vi "AssertFalse.vi"(7 "Message (\"\")":string, 8 "error in (no error)":errorcluster, 10 "Condition":bool) -> (0 "error out":errorcluster, 2 "Result":bool)   [LabVIEW 2019, in "Assertion.lvlib"]
doc: "Asserts that a condition is <B>false</B>. Does nothing if an error occurred before this node runs. Returns an error if the assertion failed. Optionally adds a message to the error message if the assertion failed."
uses:
  Assertion.lvlib
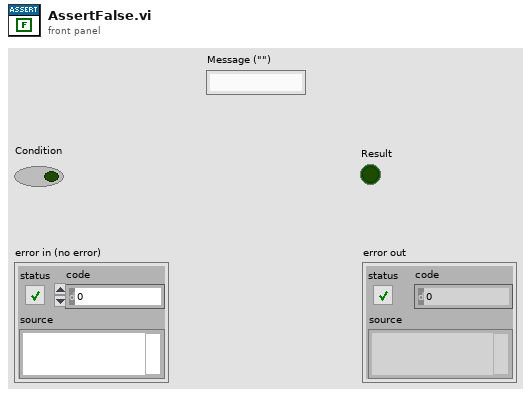
[diagram p1: front panel]
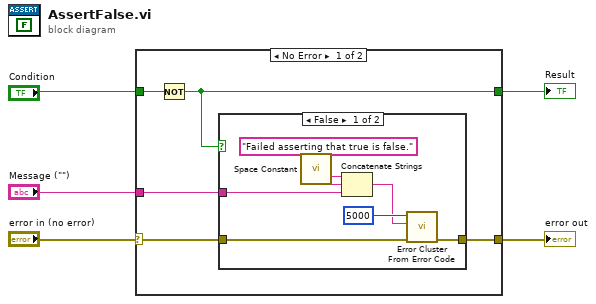
[diagram p0: block diagram]
diagram:
  n1 = case shown="No Error" "error in (no error)" {
    selector: "error in (no error)" -> [w9 w19]
    tunnel: "Condition" -> [w10 _]
    tunnel: [w7 _] -> w1
    tunnel: [w8 w19] -> w3
    tunnel: "Message (\"\")" -> [w6 _]
    frame No Error {
      n2 = Not(x=w10) -> (.not. x?=w7:bool)
      n3 = case shown="False" w7 {
        tunnel: w9 -> [w17 w18]
        tunnel: [w16 w18] -> w8
        tunnel: w6 -> [w14 _]
        frame False {
          n4 = call <vilib>:"Space Constant.vi"() -> ("String"=w13:string)
          n5 = Concatenate Strings("Failed asserting that true is false.", w13, w14) -> (w11:string)
          n6 = call <vilib>:"Error Cluster From Error Code.vi"("error in (no error)"=w17, "error message (\"\")"=w11, "error code (0)"=5000) -> ("error out"=w16:errorcluster)  [unwired: 6 in]
        }
        frame True {
        }
      }
    }
    frame Error {
    }
  }
  "error out" <- w3
  "Result" <- w1
